vi "lines_builder.vi"(7 "measure?":dbl=3.0, 10 "Config data":path, 11 "Lines data":path) -> (1 "To":dbl[](array[numeric]), 2 "From":dbl[](array[numeric]), 3 "Lines (out)":string)   [LabVIEW 2014]
uses:
  <vilib>/Utility/file.llb/Read From Spreadsheet File (DBL).vi
  <vilib>/Utility/file.llb/Read From Spreadsheet File (string).vi
panel:
  out "s? t:f":i32
  out "Boolean":bool
  out "String":string
  out "Reatances":dbl[][](array[numeric])
  out "Resistances":dbl[][](array[numeric])
  out "config":dbl[](array[numeric])
  out "Distance (miles)":dbl[](array[numeric])
  # "LINES BUILDER"
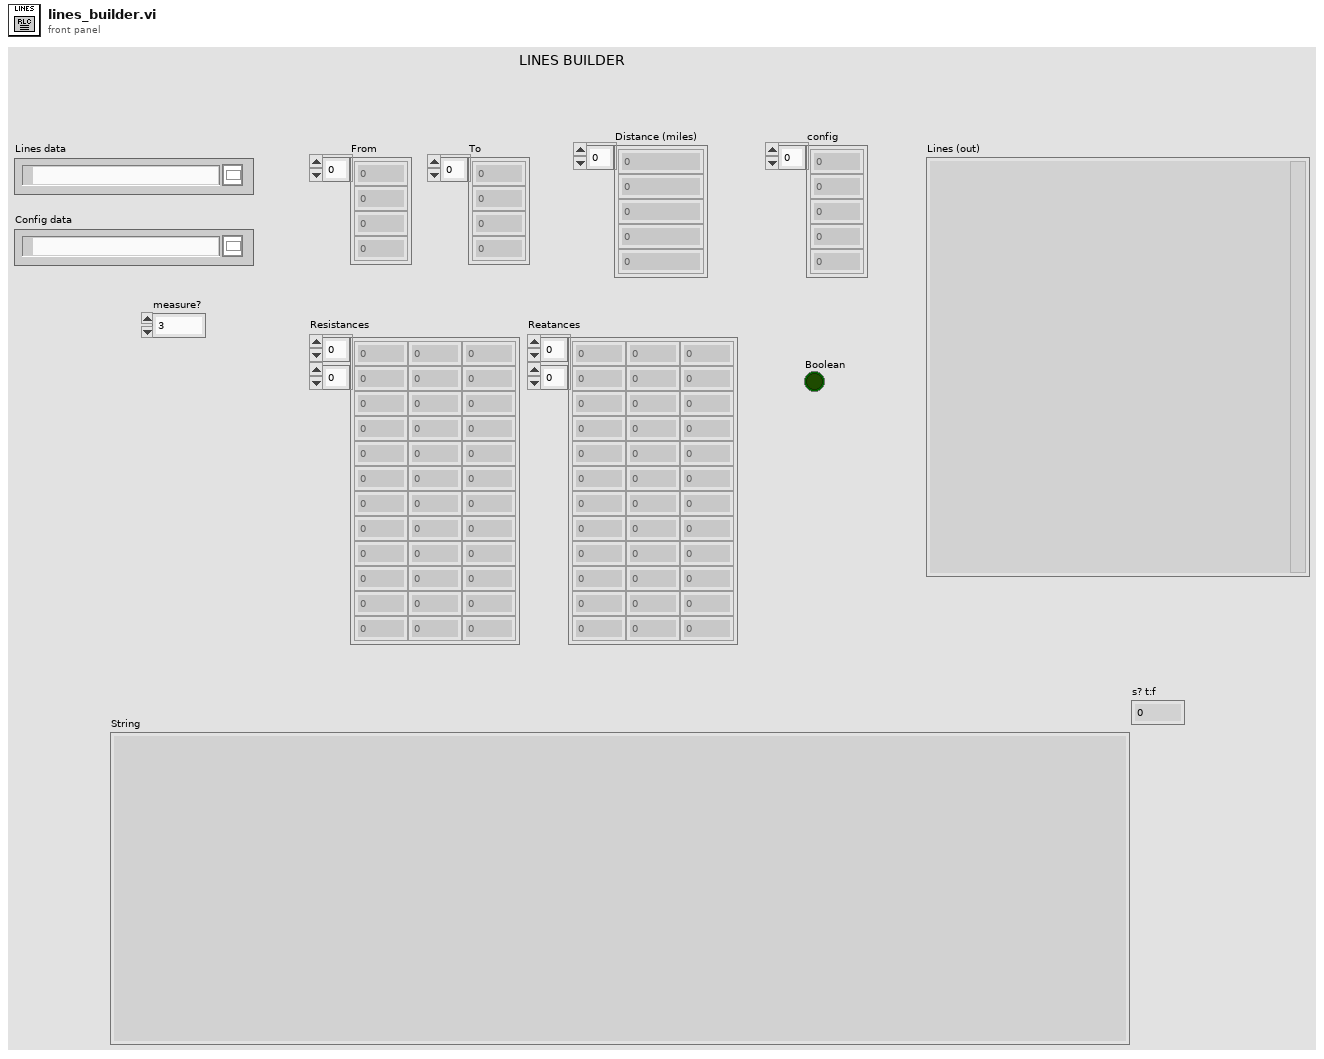
[diagram p1: front panel]
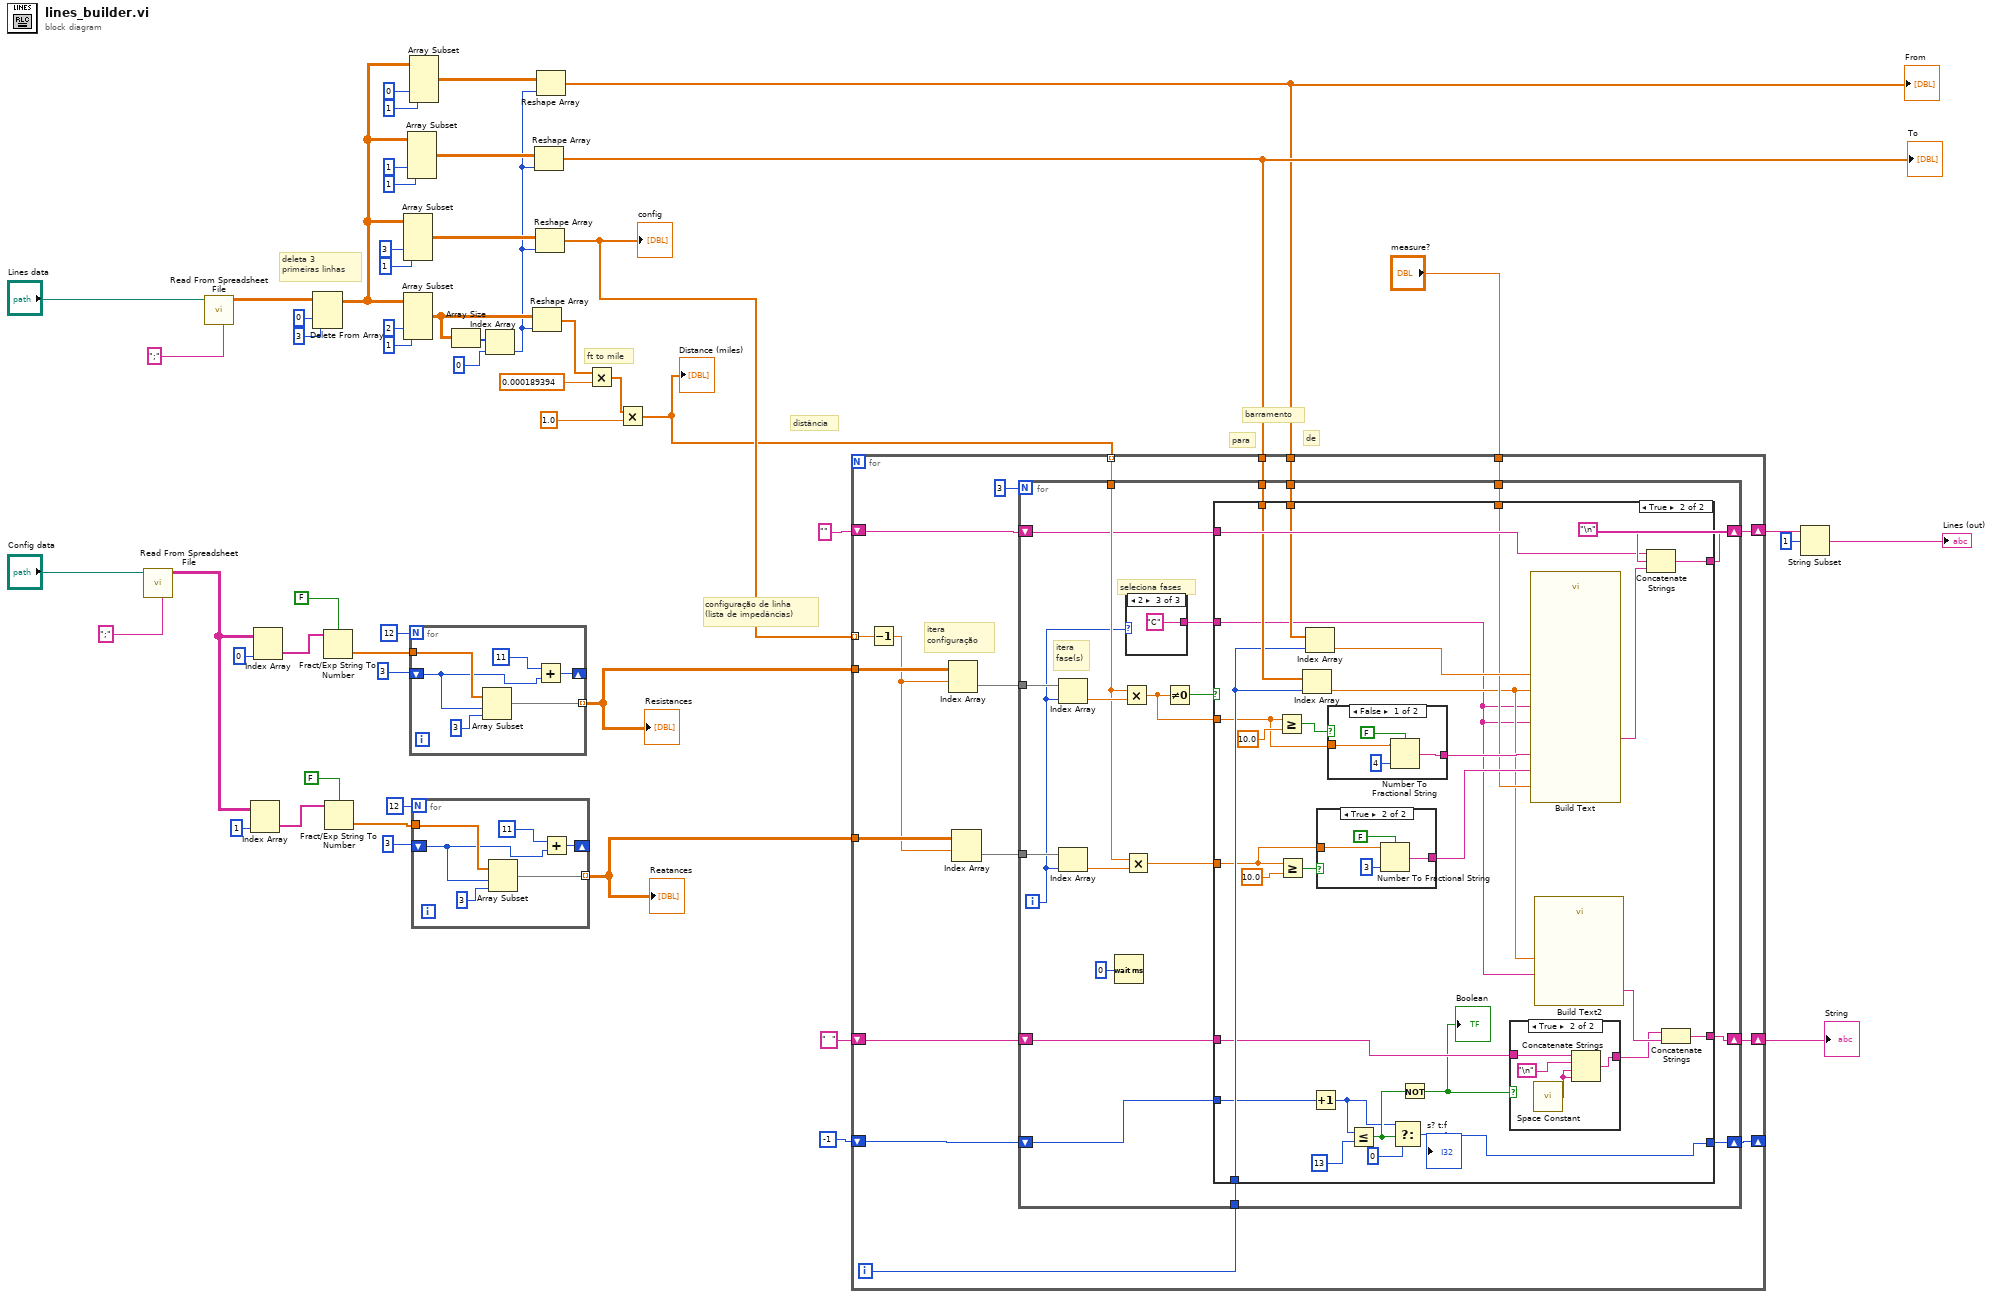
[diagram p0: block diagram]
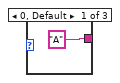
[diagram p2: hidden frame]
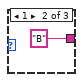
[diagram p3: hidden frame]
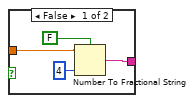
[diagram p6: hidden frame]
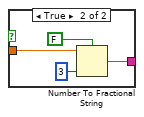
[diagram p7: hidden frame]
diagram:
  # "barramento"
  # "para"
  # "de"
  # "distância"
  # "configuração de linha \n(lista de impedâncias)"
  # "deleta 3\nprimeiras linhas"
  # "ft to mile"
  n1 = call-poly <vilib>:"Read From Spreadsheet File.vi"("delimiter (\\t)"=";" ("delimiter (\\t)"), "file path (dialog if empty)"="Config data") -> ("all rows"=w23:string[][])  [unwired: 5 in, 4 out]
  n2 = call-poly <vilib>:"Read From Spreadsheet File.vi"("delimiter (\\t)"=";" ("delimiter (\\t)"), "file path (dialog if empty)"="Lines data") -> ("all rows"=w50:dbl[][])  [unwired: 5 in, 4 out]
  n3 = Index Array(array=w23, index (col)=1 ("disabled index (col)")) -> (element=w17:string[])  [unwired: 1 in]
  n4 = Index Array(array=w23, index (col)=0 ("disabled index (col)")) -> (element=w21:string[])  [unwired: 1 in]
  n5 = Delete From Array(array=w50, length=3, index (row)=0) -> (array with subset deleted=w32:dbl[][])  [unwired: 1 in, 1 out]
  n6 = Fract/Exp String To Number(use system decimal point (T)=FALSE, string=w21) -> (number=w19:dbl[])  [unwired: 2 in, 1 out]
  n7 = Fract/Exp String To Number(use system decimal point (T)=FALSE, string=w17) -> (number=w18:dbl[])  [unwired: 2 in, 1 out]
  n8 = Array Subset(array=w32, index (col)=3 ("index"), length (col)=1 ("length")) -> (w31:dbl[][])  [unwired: 2 in]
  n9 = Array Subset(array=w32, index (col)=2 ("index"), length (col)=1 ("length")) -> (w45:dbl[][])  [unwired: 2 in]
  n10 = Array Subset(array=w32, index (col)=1 ("index"), length (col)=1 ("length")) -> (w29:dbl[][])  [unwired: 2 in]
  n11 = Array Subset(array=w32, index (col)=0 ("index"), length (col)=1 ("length")) -> (w30:dbl[][])  [unwired: 2 in]
  n12 = for {
    N: 12 -> [_]
    tunnel: w19 -> [w60]
    shift-right: [w56] -> _
    shift-left: 3 ("length") -> [w57]
    tunnel: [w55] -> w27 mode=indexing
    n13 = Array Subset(array=w60, index=w57, length=3) -> (w55:dbl[])
    n14 = Add(x=11 ("length"), y=w57) -> (x+y=w56:i32)
  }
  "Resistances" <- w27
  n15 = for {
    N: 12 -> [_]
    tunnel: w18 -> [w66]
    shift-right: [w62] -> _
    shift-left: 3 ("length") -> [w63]
    tunnel: [w61] -> w15 mode=indexing
    n16 = Array Subset(array=w66, index=w63, length=3) -> (w61:dbl[])
    n17 = Add(x=11 ("length"), y=w63) -> (x+y=w62:i32)
  }
  "Reatances" <- w15
  n18 = Array Size(array=w45) -> (size(s)=w44:i32[])
  n19 = Index Array(array=w44, index=0) -> (element=w28:i32)
  n20 = Reshape Array(w45, w28) -> (w42:dbl[])
  n21 = Reshape Array(w29, w28) -> (w13:dbl[])
  "To" <- w13
  n22 = Reshape Array(w31, w28) -> (w22:dbl[])
  "config" <- w22
  n23 = Reshape Array(w30, w28) -> (w12:dbl[])
  "From" <- w12
  n24 = Multiply(x=w42, y=0.000189394) -> (x*y=w11:dbl[])
  n25 = Multiply(x=w11, y=1.0) -> (x*y=w10:dbl[])
  "Distance (miles)" <- w10
  n26 = for {
    tunnel: w27 -> [w84]
    tunnel: w15 -> [w81]
    tunnel: w22 -> [w73] mode=indexing
    tunnel: w10 -> [w79] mode=indexing
    shift-right: [w77] -> w8
    shift-left: "" -> [w78]
    tunnel: w13 -> [w76]
    tunnel: w12 -> [w75]
    tunnel: "measure?" -> [w71]
    shift-right: [w70] -> w2
    shift-left: "  " -> [w69]
    shift-right: [w67] -> _
    shift-left: -1 -> [w68]
    i -> [w74]
    # "itera\nconfiguração"
    n27 = Decrement(x=w73) -> (x-1=w72:dbl)
    n28 = Index Array(array=w84, index (row)=w72) -> (element=w83:dbl[])  [unwired: 1 in]
    n29 = Index Array(array=w81, index (row)=w72) -> (element=w82:dbl[])  [unwired: 1 in]
    n30 = for {
      N: 3 -> [_]
      tunnel: w83 -> [w105]
      tunnel: w82 -> [w104]
      tunnel: w79 -> [w101]
      shift-right: [w98] -> w77
      shift-left: w78 -> [w99]
      tunnel: w76 -> [w93]
      tunnel: w75 -> [w92]
      tunnel: w74 -> [w91]
      tunnel: w71 -> [w90]
      shift-right: [w89] -> w70
      shift-left: w69 -> [w88]
      shift-right: [w87] -> w67
      shift-left: w68 -> [w85]
      i -> [w97]
      # "seleciona fases"
      # "itera\nfase(s)"
      n31 = Index Array(array=w105, index=w97) -> (element=w103:dbl)
      n32 = Index Array(array=w104, index=w97) -> (element=w102:dbl)
      n33 = Wait (ms)(milliseconds to wait=u32 0) -> ()  [unwired: 1 out]
      n34 = Multiply(x=w101, y=w103) -> (x*y=w95:dbl)
      n35 = Multiply(x=w101, y=w102) -> (x*y=w96:dbl)
      n36 = case shown="2" w97 {
        tunnel: ["A" "B" "C"] -> w94
        frame 0, Default {
        }
        frame 1 {
        }
        frame 2 {
        }
      }
      n37 = Not Equal To 0?(x=w95) -> (x != 0?=w100:bool)
      n38 = case shown="True" w100 {
        tunnel: w99 -> [w111 w139]
        tunnel: [w111 w140] -> w98
        tunnel: w96 -> [_ w128]
        tunnel: w95 -> [_ w130]
        tunnel: w94 -> [_ w123]
        tunnel: w93 -> [_ w137]
        tunnel: w92 -> [_ w136]
        tunnel: w91 -> [_ w134]
        tunnel: w90 -> [_ w125]
        tunnel: [w110 w122] -> w89
        tunnel: w88 -> [w110 w121]
        tunnel: w85 -> [w109 w113]
        tunnel: [w109 w117] -> w87
        frame False {
        }
        frame True {
          n39 = Greater Or Equal?(x=w130, y=10.0) -> (x >= y?=w133:bool)
          n40 = Greater Or Equal?(x=w128, y=10.0) -> (x >= y?=w127:bool)
          n41 = Index Array(array=w137, index=w134) -> (element=w124:dbl)
          n42 = Index Array(array=w136, index=w134) -> (element=w135:dbl)
          n43 = Increment(x=w113) -> (x+1=w112:i32)
          n44 = case shown="True" w127 {
            tunnel: w128 -> [w149 w153]
            tunnel: [w148 w152] -> w126
            frame False {
              n45 = Number To Fractional String(use system decimal point (T)=FALSE, number=w149, precision (6)=i16 4) -> (F-format string=w148:string)  [unwired: 1 in]
            }
            frame True {
              n46 = Number To Fractional String(use system decimal point (T)=FALSE, number=w153, precision (6)=i16 3) -> (F-format string=w152:string)  [unwired: 1 in]
            }
          }
          n47 = case shown="False" w133 {
            tunnel: w130 -> [w157 w161]
            tunnel: [w156 w160] -> w129
            frame False {
              n48 = Number To Fractional String(use system decimal point (T)=FALSE, number=w157, precision (6)=i16 4) -> (F-format string=w156:string)  [unwired: 1 in]
            }
            frame True {
              n49 = Number To Fractional String(use system decimal point (T)=FALSE, number=w161, precision (6)=i16 3) -> (F-format string=w160:string)  [unwired: 1 in]
            }
          }
          n50 = Less Or Equal?(x=w112, y=13 ("x")) -> (x <= y?=w116:bool)
          n51 = Select(t=w112, s=w116, f=0) -> (s? t:f=w117:i32)
          "s? t:f" <- w117
          n52 = Not(x=w116) -> (.not. x?=w118:bool)
          "Boolean" <- w118
          n53 = case shown="True" w118 {
            tunnel: w121 -> [w142 w143]
            tunnel: [w142 w145] -> w114
            frame False {
            }
            frame True {
              n54 = call <vilib>:"Space Constant.vi"() -> ("String"=w144:string)
              n55 = Concatenate Strings(w143, "\n", w144, w144) -> (w145:string)
            }
          }
          n56 = call "Build Text"("fase_out"=w123, "reatancia"=w126, "de"=w135, "fase_in"=w123, "para"=w124, "resistencia"=w129, "measure"=w125) -> ("Result"=w138:string)  [unwired: 7 in, 1 out]
          n57 = call "Build Text2"("node"=w124, "phase"=w123) -> ("Result"=w115:string)  [unwired: 12 in, 1 out]
          n58 = Concatenate Strings(w139, "\n", w138) -> (w140:string)
          n59 = Concatenate Strings(w114, w115) -> (w122:string)
        }
      }
    }
  }
  "String" <- w2
  n60 = String Subset(string=w8, offset (0)=1) -> (substring=→"Lines (out)":string)  [unwired: 1 in]
